vi "Main program.vi"() -> ()   [LabVIEW 2015]
doc: "Use this template to build a standard state machine design pattern. Each state executes code and determines which state to transition to. Contrast this design pattern with the User Interface Event Handler pattern, in which code executes in response to user actions. Contrast this design pattern also with the Queued Message Handler pattern, in which each message handling code can queue zero or more new messages.\nNote: This template does not contain the most recent programming guidelines recommended by National Instruments. For a complete, project-based implementation of the Standard State Machine pattern, use the Create Project dialog box instead of this template."
uses:
  StateMachineStates.ctl
  <vilib>/Analysis/6fits.llb/Curve Fitting Criteria.ctl
  <vilib>/Utility/file.llb/Read From Spreadsheet File (DBL).vi
  <vilib>/Analysis/NI_AALPro.lvlib
panel:
  out "Galv. cal. data":dbl[][](array[numeric])
  out "Galvanostatic":bool
  out "Potentiostatic":bool
  out "DAC calibration data":dbl[][](array[numeric]) format="%0.3f"
  out "Cell on (checkbox)":bool
  out "Current (µA)":dbl format="%.3f"
  in  "Stop button":bool
  out "Voltage (V)":dbl format="%.5f"
  in  "Tab Control":T1(tab)
  in  "Cell on (button)":bool
  in  "Mode":string(combo)="Potentiostatic"
  in  "Current Range":string(combo)="2"
  out "Serial Number":string
  out "Model Name":string
  out "Manufacturer Name":string
  out "Calibrated":bool
  in  "Load DAC calibration":bool
  in  "Scan DAC codes":bool
  out "Code":u16
  in  "DAC output (V)":dbl(slide) scale=0.0..4.8
  out "Config. byte":u8 format="%02x"
  out "Config. byte":u8 format="%02x"
  in  "Calibration factor":dbl=1.0 min=1.0 max=1.0
  in  "ADC CH2 - Current":bool=TRUE
  in  "Bit Depth selection 2":enum32{"CH1", "CH2", "CH2 2", "CH2 3"}(radio)=enum."CH2 3"
  in  "Calibration factor":dbl=3.0
  in  "ADC CH1 - Voltage":bool=TRUE
  in  "Bit Depth selection 1":enum32{"CH1", "CH2", "CH2 2", "CH2 3"}(radio)=enum."CH2 2"
  out "Calibrated 2":bool
  in  "Load galv. calibration":bool
  in  "Calibrate galvanostatic":bool
  in  "VISA resource":refnum<visa-resource-name>
  in  "Auto bit depth":bool
  out "CV graph":cluster{dbl[], dbl[]}(graph)
  in  "Start CV":bool
  in  "Lower bound (V)":dbl=1.0
  in  "Scan rate (mV/s)":dbl=20.0
  in  "Stop CV":bool
  in  "Start potential (V)":dbl=1.0
  in  "Stop potential (V)":dbl=3.0
  in  "Number of cycles":u16
  in  "Upper bound (V)":dbl=3.0
  in  "Copy OCP":bool
  in  "Export filename":path
  in  "Auto range":bool
  out "Calculated capacity values (µAh)":dbl[](array[numeric]) format="%#.4f"
  out "Discharge capacity (µAh)":dbl
  out "Charge capacity (µAh)":dbl
  out "Current half cycle":i32
  in  "Start CC":bool
  in  "Stop CC":bool
  in  "Export filename":path
  in  "Number of\nhalf cycles":u16=3 min=1 step=1
  in  "Copy negative":bool
  in  "Discharge\ncurrent (µA)":dbl=1.0
  in  "Charge\ncurrent (µA)":dbl=1.0
  out "CC ch/disch graph":cluster{dbl[], dbl[]}(graph)
  in  "Upper limit (V)":dbl=3.0
  in  "Lower limit (V)":dbl=1.0
  # "Interface"
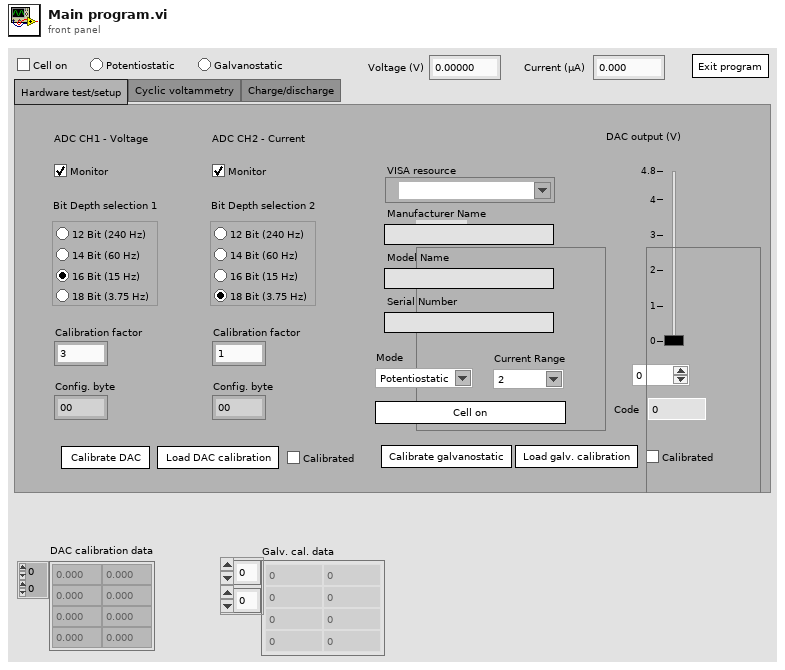
[diagram p1: front panel]
types:
  T1 = enum32{"Hardware test/setup", "Cyclic voltammetry", "Charge/discharge"}
  T2 = typedef "StateMachineStates.ctl" = enum16{"Initialize", "Wait for input", "Perform CV scan", "CC charge/discharge", "Scan DAC codes", "Calibrate galvanostatic", "Stop"}
  T3 = enum16{"open", "replace", "create", "open or create", "replace or create", "replace or create with confirmation"}
  T4 = typedef "NI_AALPro.lvlib/Curve Fitting Criteria.ctl" = u16
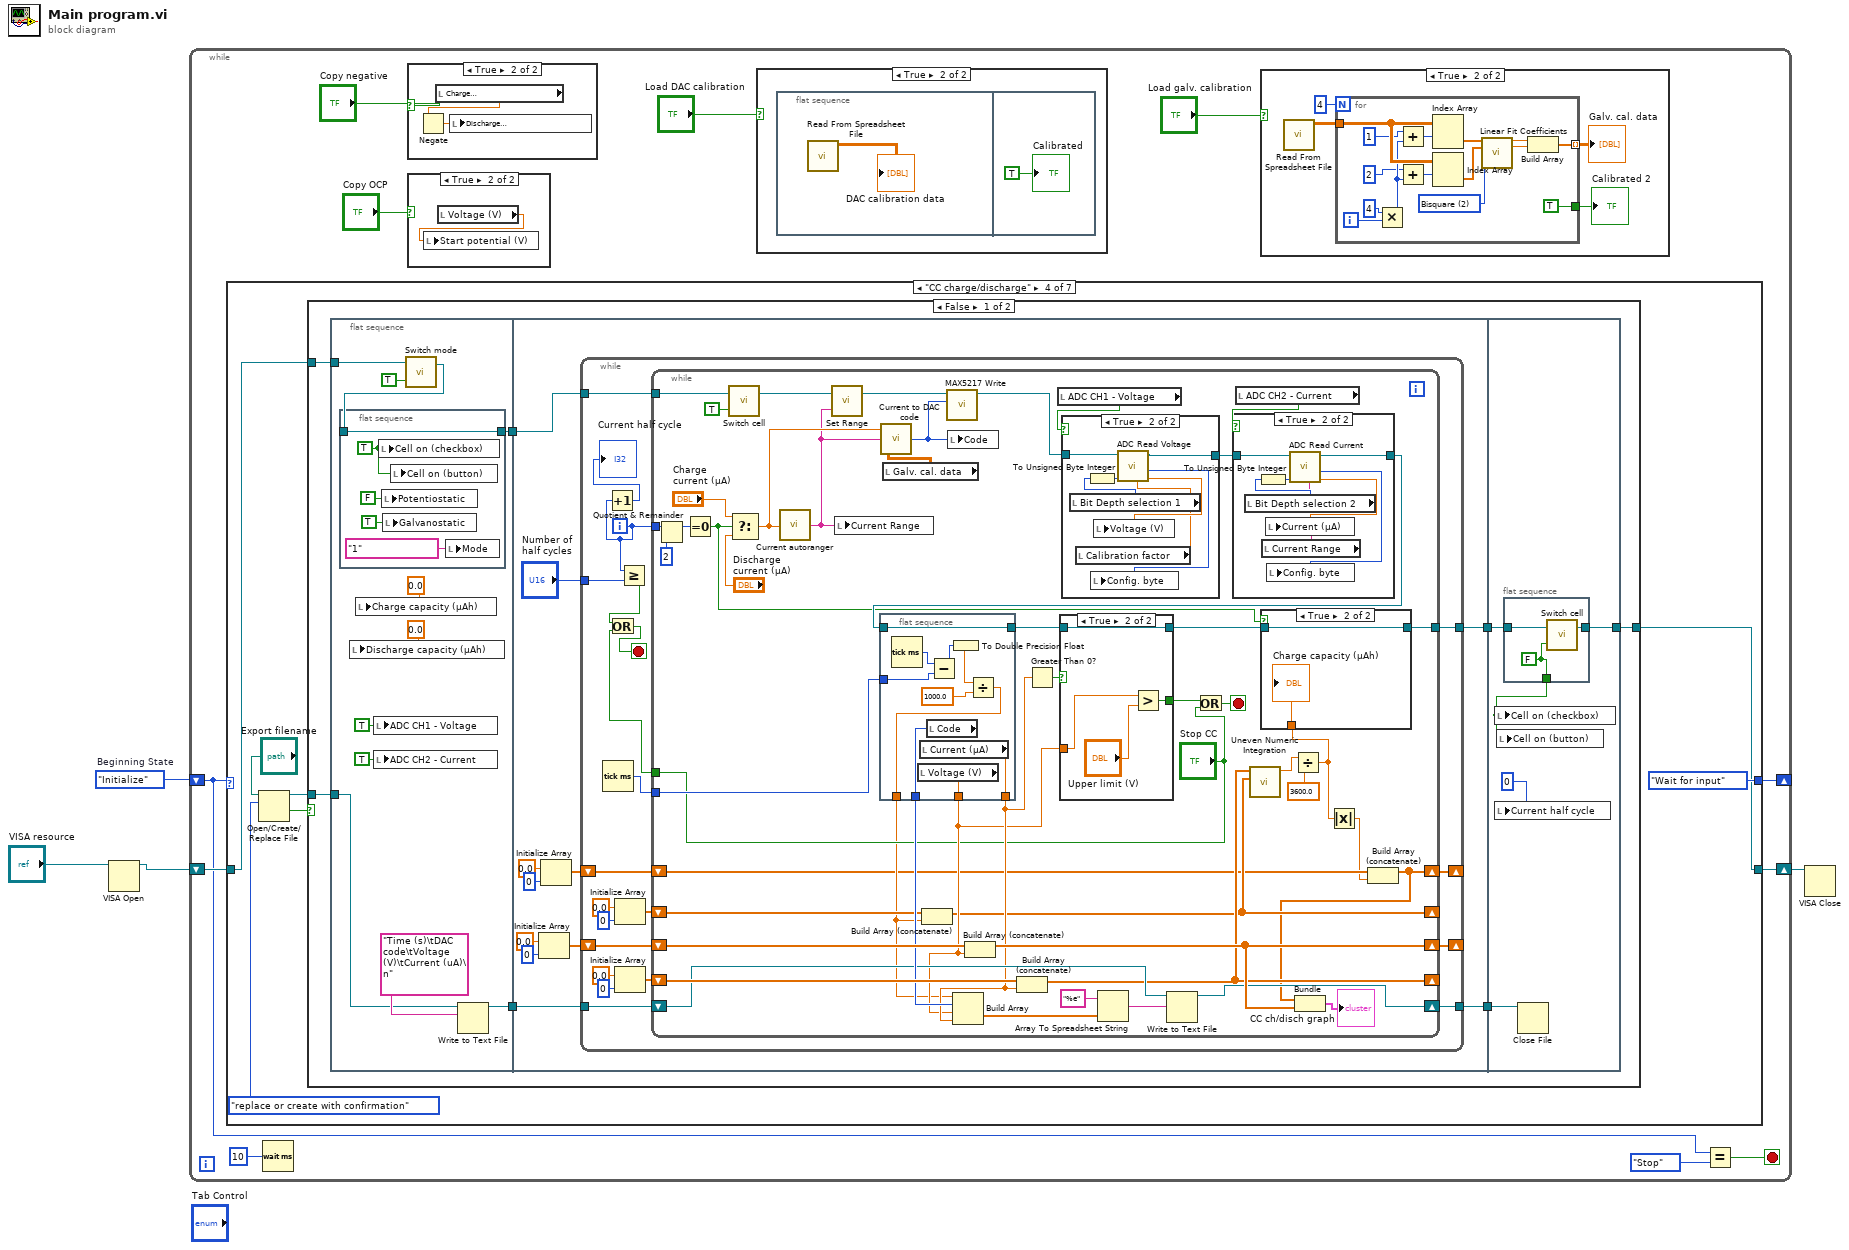
[diagram p0: block diagram]
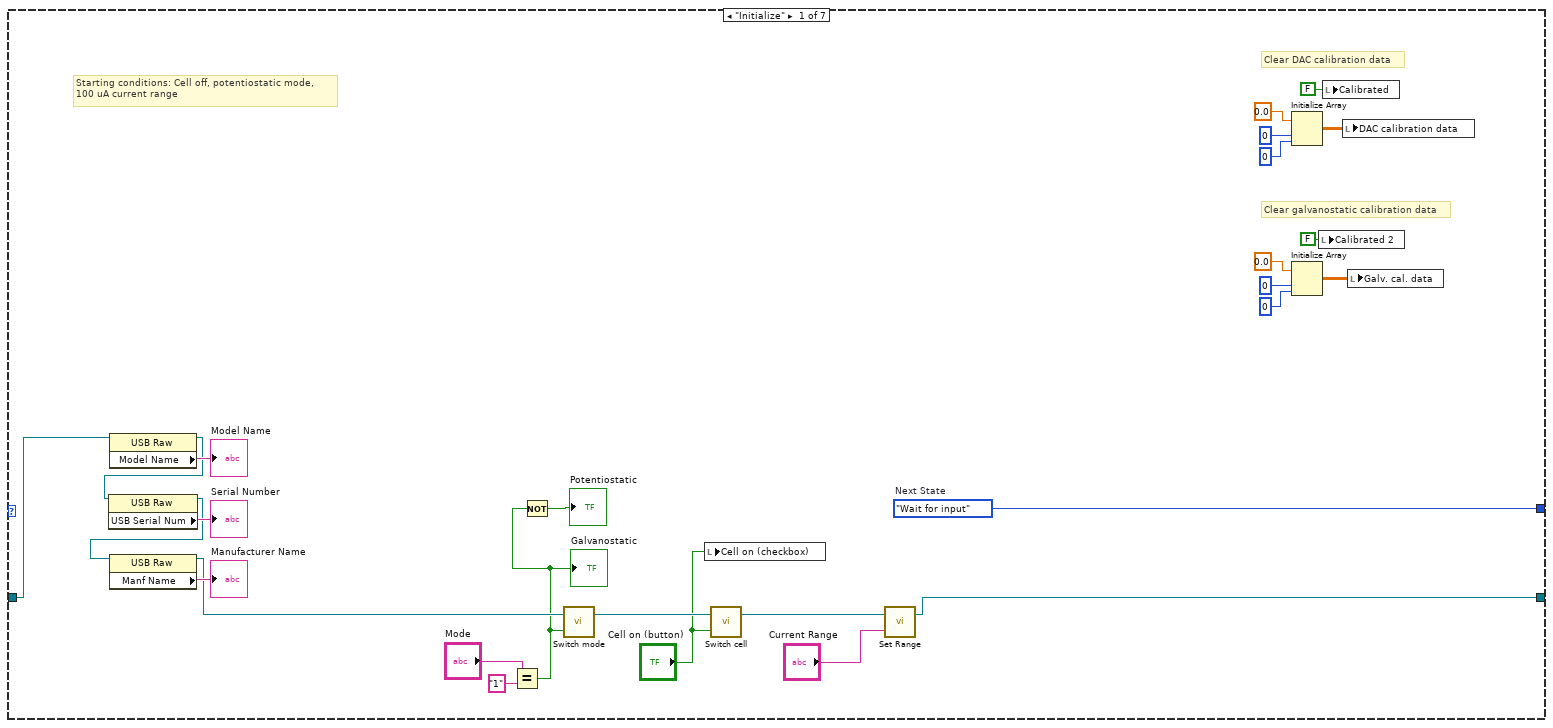
[diagram p6: hidden frame]
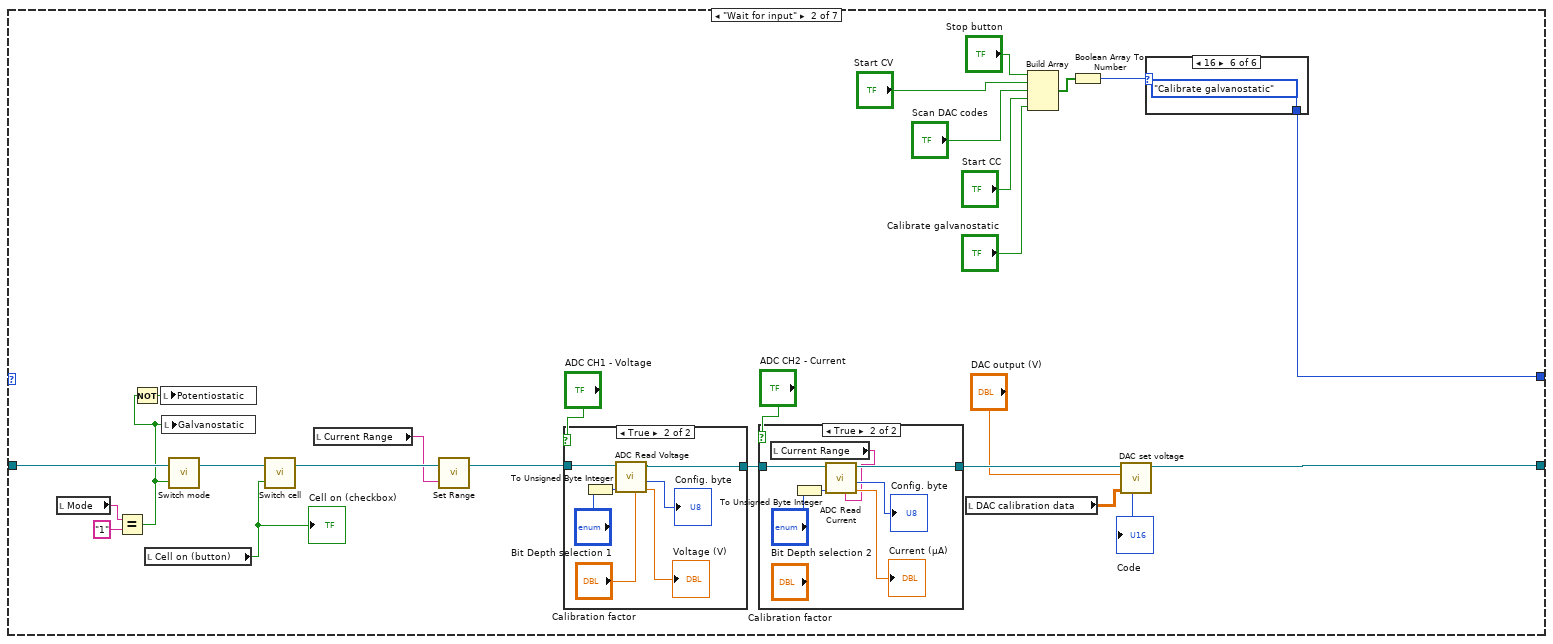
[diagram p7: hidden frame]
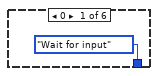
[diagram p10: hidden frame]
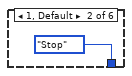
[diagram p11: hidden frame]
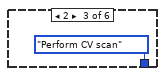
[diagram p12: hidden frame]
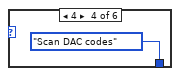
[diagram p13: hidden frame]
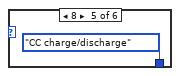
[diagram p14: hidden frame]
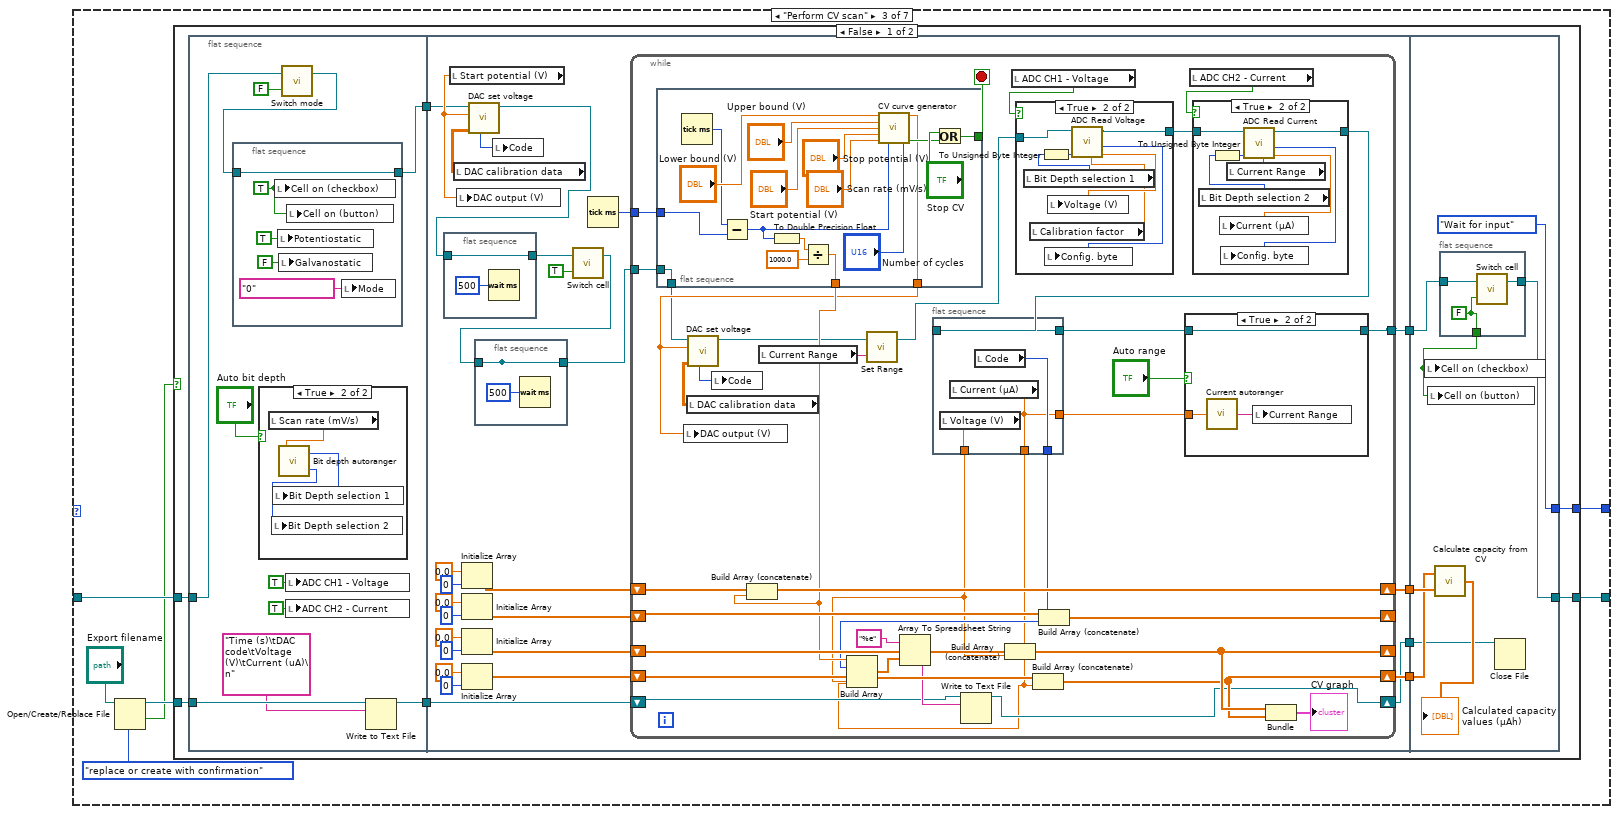
[diagram p15: hidden frame]
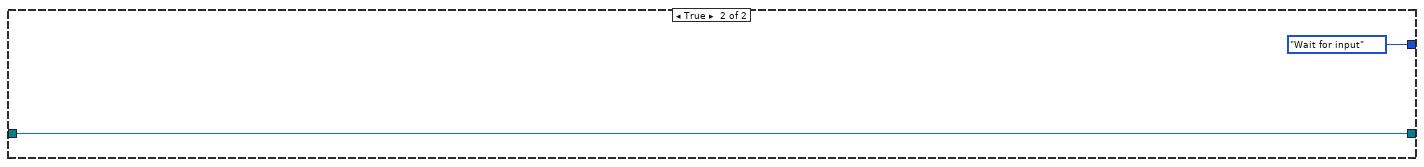
[diagram p20: hidden frame]
diagram:
  w4 = StateMachineStates."Initialize"  # Beginning State
  n1 = VISA Open(VISA resource name="VISA resource") -> (VISA resource name=w1:refnum<visa-resource-name>)  [unwired: 4 in, 1 out]
  n2 = while {
    shift-right: [w14] -> _
    shift-left: w4 -> [w10]
    shift-right: [w11] -> w3
    shift-left: w1 -> [w12]
    stop <- w9 stop-if-true
    n3 = case shown="\"CC charge/discharge\"" w10 {
      tunnel: [w66 w90 w120 StateMachineStates."Wait for input" ("Next State") StateMachineStates."Wait for input" ("Next State") StateMachineStates."Wait for input" ("Next State") StateMachineStates."Stop" ("Next State")] -> w14
      tunnel: w12 -> [w52 w75 w121 w273 w430 w490 w580]
      tunnel: [w40 w83 w119 w271 w429 w491 w580] -> w11
      frame "Initialize" {
        w66 = StateMachineStates."Wait for input"  # Next State
        # "Clear galvanostatic calibration data"
        # "Clear DAC calibration data"
        # "Starting conditions: Cell off, potentiostatic mode,\n100 uA current range"
        n4 = property class="USB Raw"(reference=w52) -> (reference out=w51:refnum<visa-resource-name>, "Model Name"=→"Model Name":string)  [unwired: 1 in, 1 out]
        n5 = property class="USB Raw"(reference=w51) -> (reference out=w50:refnum<visa-resource-name>, "USB Serial Num"=→"Serial Number":string)  [unwired: 1 in, 1 out]
        n6 = property class="USB Raw"(reference=w50) -> (reference out=w48:refnum<visa-resource-name>, "Manf Name"=→"Manufacturer Name":string)  [unwired: 1 in, 1 out]
        n7 = Equal?(x="Mode", y="1") -> (x = y?=w42:bool)
        "Galvanostatic" <- w42
        n8 = Not(x=w42) -> (.not. x?=→"Potentiostatic":bool)
        n9 = call "Switch mode.vi"("Galvanostatic"=w42, "VISA Refnum in"=w48) -> ("VISA Refnum out"=w45:refnum<visa-resource-name>)  [unwired: 1 in]
        n10 = local write "Cell on (checkbox)"("Cell on (button)") -> ()
        n11 = call "Switch cell.vi"("Boolean"="Cell on (button)", "VISA Refnum in"=w45) -> ("VISA Refnum out"=w44:refnum<visa-resource-name>)  [unwired: 1 in]
        n12 = call "Set Range.vi"("Range #"="Current Range", "VISA Refnum in"=w44) -> ("VISA Refnum out"=w40:refnum<visa-resource-name>)  [unwired: 1 in]
        n13 = Initialize Array(0.0 ("element"), 0 ("dimension size"), 0 ("dimension size")) -> (w62:dbl[][])
        n14 = Initialize Array(0.0 ("element"), 0 ("dimension size"), 0 ("dimension size")) -> (w59:dbl[][])
        n15 = local write "Calibrated 2"(FALSE ("Calibrated")) -> ()
        n16 = local write "Calibrated"(FALSE ("Calibrated")) -> ()
        n17 = local write "DAC calibration data"(w62) -> ()
        n18 = local write "Galv. cal. data"(w59) -> ()
      }
      frame "Wait for input" {
        n19 = local read "Mode"() -> (w71:string)
        n20 = Equal?(x=w71, y="1") -> (x = y?=w69:bool)
        n21 = Not(x=w69) -> (.not. x?=w70:bool)
        n22 = local read "Cell on (button)"() -> (w68:bool)
        "Cell on (checkbox)" <- w68
        n23 = local write "Potentiostatic"(w70) -> ()
        n24 = local write "Galvanostatic"(w69) -> ()
        n25 = call "Switch mode.vi"("Galvanostatic"=w69, "VISA Refnum in"=w75) -> ("VISA Refnum out"=w74:refnum<visa-resource-name>)  [unwired: 1 in]
        n26 = call "Switch cell.vi"("Boolean"=w68, "VISA Refnum in"=w74) -> ("VISA Refnum out"=w73:refnum<visa-resource-name>)  [unwired: 1 in]
        n27 = local read "Current Range"() -> (w67:string)
        n28 = call "Set Range.vi"("Range #"=w67, "VISA Refnum in"=w73) -> ("VISA Refnum out"=w72:refnum<visa-resource-name>)  [unwired: 1 in]
        n29 = case shown="True" "ADC CH1 - Voltage" {
          tunnel: [w101 w108] -> w86
          tunnel: w72 -> [w101 w107]
          frame False {
          }
          frame True {
            n30 = To Unsigned Byte Integer(number="Bit Depth selection 1") -> (unsigned 8bit integer=w102:u8)
            n31 = call "ADC Read Voltage.vi"("Calibration factor"="Calibration factor", "Bit depth"=w102, "VISA Refnum in"=w107) -> ("Voltage in V"=→"Voltage (V)":dbl, "Configuration byte"=→"Config. byte":u8, "VISA Refnum out"=w108:refnum<visa-resource-name>)  [unwired: 6 in]
          }
        }
        n32 = case shown="True" "ADC CH2 - Current" {
          tunnel: w86 -> [w93 w100]
          tunnel: [w93 w99] -> w84
          frame False {
          }
          frame True {
            n33 = local read "Current Range"() -> (w94:string)
            n34 = To Unsigned Byte Integer(number="Bit Depth selection 2") -> (unsigned 8bit integer=w97:u8)
            n35 = call "ADC Read Current.vi"("Range"=w94, "Bit depth"=w97, "VISA Refnum in"=w100) -> ("Current in uA"=→"Current (µA)":dbl, "Configuration byte"=→"Config. byte":u8, "VISA Refnum out"=w99:refnum<visa-resource-name>)  [unwired: 6 in]
          }
        }
        n36 = local read "DAC calibration data"() -> (w79:dbl[][])
        n37 = Build Array("Stop button", "Start CV", "Scan DAC codes", "Start CC", "Calibrate galvanostatic") -> (w92:bool[])
        n38 = Boolean Array To Number(Boolean array=w92) -> (number=w91:u32)
        n39 = call "DAC set voltage.vi"("Calibration array"=w79, "DAC output (V)"="DAC output (V)", "VISA Refnum in"=w84) -> ("VISA Refnum out"=w83:refnum<visa-resource-name>, "Output code"=→"Code":u16)  [unwired: 7 in]
        n40 = case shown="16" w91 {
          tunnel: [StateMachineStates."Wait for input" ("f") StateMachineStates."Stop" ("f") StateMachineStates."Perform CV scan" ("f") StateMachineStates."Scan DAC codes" ("f") StateMachineStates."CC charge/discharge" ("f") StateMachineStates."Calibrate galvanostatic" ("f")] -> w90
          frame 0 {
          }
          frame 1, Default {
          }
          frame 2 {
          }
          frame 4 {
          }
          frame 8 {
          }
          frame 16 {
          }
        }
      }
      frame "Perform CV scan" {
        n41 = Open/Create/Replace File(file path (use dialog)="Export filename", operation (0:open)=T3."replace or create with confirmation") -> (refnum out=w116:refnum<file>, cancelled=w115:bool)  [unwired: 4 in, 1 out]
        n42 = case shown="False" w115 {
          tunnel: w121 -> [w128 w270]
          tunnel: [w123 StateMachineStates."Wait for input" ("Next State")] -> w120
          tunnel: [w127 w270] -> w119
          tunnel: w116 -> [w126 _]
          frame False {
            n43 = flat-sequence {
              tunnel: w128 -> [w140]
              tunnel: [w138] -> w131
              tunnel: w126 -> [w134]
              tunnel: [w133] -> w130
              tunnel: w131 -> [w155]
              tunnel: [w163] -> w129
              tunnel: w130 -> [w162]
              tunnel: [w161] -> w125
              tunnel: [w160] -> w124
              tunnel: [w159] -> w122
              tunnel: [w265] -> w127
              tunnel: w129 -> [w264]
              tunnel: w125 -> [w261]
              tunnel: w124 -> [w262]
              tunnel: [StateMachineStates."Wait for input" ("Next State")] -> w123
              tunnel: w122 -> [w259]
              frame #0 {
                n44 = flat-sequence {
                  tunnel: w139 -> [w149]
                  tunnel: [w149] -> w138
                  frame #0 {
                    w146 = TRUE ("Boolean")
                    n45 = local write "Cell on (checkbox)"(w146) -> ()
                    n46 = local write "Potentiostatic"(TRUE ("Potentiostatic")) -> ()
                    n47 = local write "Galvanostatic"(FALSE ("Galvanostatic")) -> ()
                    n48 = local write "Cell on (button)"(w146) -> ()
                    n49 = local write "Mode"("0" ("Mode")) -> ()
                  }
                }
                n50 = case shown="True" "Auto bit depth" {
                  frame False {
                  }
                  frame True {
                    n51 = local read "Scan rate (mV/s)"() -> (w144:dbl)
                    n52 = call "Bit depth autoranger.vi"("Scan rate (mV/s)"=w144) -> ("I bit depth setting"=w142:u8, "V bit depth setting"=w143:u8)  [unwired: 1 in]
                    n53 = local write "Bit Depth selection 2"(w142) -> ()
                    n54 = local write "Bit Depth selection 1"(w143) -> ()
                  }
                }
                n55 = call "Switch mode.vi"("Galvanostatic"=FALSE, "VISA Refnum in"=w140) -> ("VISA Refnum out"=w139:refnum<visa-resource-name>)  [unwired: 1 in]
                n56 = local write "ADC CH1 - Voltage"(TRUE ("ADC CH1 - Voltage")) -> ()
                n57 = local write "ADC CH2 - Current"(TRUE ("ADC CH2 - Current")) -> ()
                n58 = Write to Text File(file (use dialog)=w134, text="Time (s)\tDAC code\tVoltage (V)\tCurrent (uA)\n") -> (refnum out=w133:refnum<file>)  [unwired: 2 in, 2 out]
              }
              frame #1 {
                n59 = flat-sequence {
                  tunnel: [w179] -> w152
                  tunnel: w154 -> [w179]
                  frame #0 {
                    n60 = Wait (ms)(milliseconds to wait=u32 500) -> ()  [unwired: 1 out]
                  }
                }
                n61 = local read "Start potential (V)"() -> (w156:dbl)
                n62 = local read "DAC calibration data"() -> (w157:dbl[][])
                n63 = local write "DAC output (V)"(w156) -> ()
                n64 = Initialize Array(0.0 ("element"), 0 ("dimension size")) -> (w167:dbl[])
                n65 = Initialize Array(0.0 ("element"), 0 ("dimension size")) -> (w164:dbl[])
                n66 = Initialize Array(0.0 ("element"), 0 ("dimension size")) -> (w175:dbl[])
                n67 = Initialize Array(0.0 ("element"), 0 ("dimension size")) -> (w172:dbl[])
                n68 = call "DAC set voltage.vi"("Calibration array"=w157, "DAC output (V)"=w156, "VISA Refnum in"=w155) -> ("VISA Refnum out"=w154:refnum<visa-resource-name>, "Output code"=w158:u16)  [unwired: 7 in]
                n69 = flat-sequence {
                  tunnel: [w177] -> _
                  tunnel: w151 -> [w177]
                  tunnel: [w177] -> w150
                  frame #0 {
                    n70 = Wait (ms)(milliseconds to wait=u32 500) -> ()  [unwired: 1 out]
                  }
                }
                n71 = local write "Code"(w158) -> ()
                n72 = call "Switch cell.vi"("Boolean"=TRUE, "VISA Refnum in"=w152) -> ("VISA Refnum out"=w151:refnum<visa-resource-name>)  [unwired: 1 in]
                n73 = Tick Count (ms)() -> (millisecond timer value=w176:u32)
                n74 = while {
                  tunnel: w176 -> [w208]
                  tunnel: w150 -> [w204]
                  tunnel: [w189] -> w163
                  shift-right: [w214] -> _
                  shift-left: w175 -> [w216]
                  shift-right: [w213] -> w161
                  shift-left: w172 -> [w215]
                  shift-right: [w210] -> w160
                  shift-left: w167 -> [w209]
                  shift-right: [w203] -> _
                  shift-left: w164 -> [w202]
                  shift-right: [w191] -> w159
                  shift-left: w162 -> [w192]
                  stop <- w211 stop-if-true
                  n75 = flat-sequence {
                    tunnel: [w241] -> w211
                    tunnel: w208 -> [w231]
                    tunnel: [w227] -> w196
                    tunnel: w204 -> [w225]
                    tunnel: [w226] -> w184
                    tunnel: [w225] -> w183
                    frame #0 {
                      n76 = Tick Count (ms)() -> (millisecond timer value=w232:u32)
                      n77 = Subtract(x=w232, y=w231) -> (x-y=w229:u32)
                      n78 = To Double Precision Float(number=w229) -> (double precision float=w228:dbl)
                      n79 = Divide(x=w228, y=1000.0) -> (x/y=w227:dbl)
                      n80 = call "CV curve generator.vi"("Lower bound (V)"="Lower bound (V)", "Upper bound (V)"="Upper bound (V)", "Start potential (V)"="Start potential (V)", "Stop potential (V)"="Stop potential (V)", "Scan rate (mV/s)"="Scan rate (mV/s)", "Time (ms)"=w229, "Number of cycles"="Number of cycles") -> ("Actual potential"=w226:dbl, "End"=w233:bool)  [unwired: 7 in]
                      n81 = Or(x="Stop CV", y=w233) -> (x .or. y?=w241:bool)
                    }
                  }
                  n82 = local write "DAC output (V)"(w184) -> ()
                  n83 = local read "DAC calibration data"() -> (w199:dbl[][])
                  n84 = call "DAC set voltage.vi"("Calibration array"=w199, "DAC output (V)"=w184, "VISA Refnum in"=w183) -> ("VISA Refnum out"=w182:refnum<visa-resource-name>, "Output code"=w200:u16)  [unwired: 7 in]
                  n85 = local write "Code"(w200) -> ()
                  n86 = Build Array (concatenate)(w209, w196) -> (w210:dbl[])
                  n87 = local read "Current Range"() -> (w185:string)
                  n88 = Build Array(w196, w195, w194, w186) -> (w197:dbl[])
                  n89 = call "Set Range.vi"("Range #"=w185, "VISA Refnum in"=w182) -> ("VISA Refnum out"=w181:refnum<visa-resource-name>)  [unwired: 1 in]
                  n90 = Array To Spreadsheet String(array=w197, 3:"%e" ("format string")) -> (spreadsheet string=w193:string)  [unwired: 1 out]
                  n91 = flat-sequence {
                    tunnel: w201 -> [w222]
                    tunnel: [w224] -> w194
                    tunnel: [w221] -> w186
                    tunnel: [w223] -> w195
                    tunnel: [w222] -> w190
                    tunnel: [w221] -> w187
                    frame #0 {
                      n92 = local read "Voltage (V)"() -> (w224:dbl)
                      n93 = local read "Current (µA)"() -> (w221:dbl)
                      n94 = local read "Code"() -> (w223:u16)
                    }
                  }
                  n95 = Write to Text File(file (use dialog)=w192, text=w193) -> (refnum out=w191:refnum<file>)  [unwired: 2 in, 2 out]
                  n96 = Build Array (concatenate)(w216, w194) -> (w214:dbl[])
                  n97 = local read "ADC CH1 - Voltage"() -> (w206:bool)
                  n98 = case shown="True" w206 {
                    tunnel: [w250 w257] -> w207
                    tunnel: w181 -> [w250 w256]
                    frame False {
                    }
                    frame True {
                      n99 = local read "Bit Depth selection 1"() -> (w254:enum32{"CH1", "CH2", "CH2 2", "CH2 3"})
                      n100 = local read "Calibration factor"() -> (w252:dbl)
                      n101 = To Unsigned Byte Integer(number=w254) -> (unsigned 8bit integer=w255:u8)
                      n102 = call "ADC Read Voltage.vi"("Calibration factor"=w252, "Bit depth"=w255, "VISA Refnum in"=w256) -> ("Voltage in V"=w253:dbl, "Configuration byte"=w251:u8, "VISA Refnum out"=w257:refnum<visa-resource-name>)  [unwired: 6 in]
                      n103 = local write "Config. byte"(w251) -> ()
                      n104 = local write "Voltage (V)"(w253) -> ()
                    }
                  }
                  n105 = Build Array (concatenate)(w215, w186) -> (w213:dbl[])
                  n106 = Build Array (concatenate)(w202, w195) -> (w203:dbl[])
                  n107 = case shown="True" "Auto range" {
                    tunnel: w190 -> [w217 w220]
                    tunnel: [w217 w220] -> w189
                    tunnel: w187 -> [_ w219]
                    frame False {
                    }
                    frame True {
                      n108 = call "Current autoranger.vi"("Current (µA)"=w219) -> ("Range"=w218:string)
                      n109 = local write "Current Range"(w218) -> ()
                    }
                  }
                  n110 = local read "ADC CH2 - Current"() -> (w205:bool)
                  n111 = case shown="True" w205 {
                    tunnel: w207 -> [w242 w249]
                    tunnel: [w242 w248] -> w201
                    frame False {
                    }
                    frame True {
                      n112 = local read "Bit Depth selection 2"() -> (w246:enum32{"CH1", "CH2", "CH2 2", "CH2 3"})
                      n113 = To Unsigned Byte Integer(number=w246) -> (unsigned 8bit integer=w247:u8)
                      n114 = local read "Current Range"() -> (w243:string)
                      n115 = call "ADC Read Current.vi"("Range"=w243, "Bit depth"=w247, "VISA Refnum in"=w249) -> ("Current in uA"=w245:dbl, "Configuration byte"=w244:u8, "VISA Refnum out"=w248:refnum<visa-resource-name>)  [unwired: 6 in]
                      n116 = local write "Current (µA)"(w245) -> ()
                      n117 = local write "Config. byte"(w244) -> ()
                    }
                  }
                  n118 = Bundle(w214, w213) -> (→"CV graph":cluster{dbl[], dbl[]})  [unwired: 1 in]
                }
              }
              frame #2 {
                n119 = local write "Cell on (checkbox)"(w258) -> ()
                n120 = local write "Cell on (button)"(w258) -> ()
                n121 = call "Calculate capacity from CV.vi"("t values"=w262, "I values"=w261) -> ("Capacity values"=→"Calculated capacity values (µAh)":dbl[])  [unwired: 1 in]
                n122 = flat-sequence {
                  tunnel: w264 -> [w268]
                  tunnel: [w267] -> w265
                  tunnel: [w266] -> w258
                  frame #0 {
                    w266 = FALSE ("Boolean")
                    n123 = call "Switch cell.vi"("Boolean"=w266, "VISA Refnum in"=w268) -> ("VISA Refnum out"=w267:refnum<visa-resource-name>)  [unwired: 1 in]
                  }
                }
                n124 = Close File(refnum=w259) -> ()  [unwired: 1 in, 2 out]
              }
            }
          }
          frame True {
          }
        }
      }
      frame "CC charge/discharge" {
        n125 = Open/Create/Replace File(file path (use dialog)="Export filename", operation (0:open)=T3."replace or create with confirmation") -> (refnum out=w272:refnum<file>, cancelled=w274:bool)  [unwired: 4 in, 1 out]
        n126 = case shown="False" w274 {
          tunnel: w273 -> [w284 w428]
          tunnel: w272 -> [w283 _]
          tunnel: [w279 w428] -> w271
          frame False {
            n127 = flat-sequence {
              tunnel: w284 -> [w294]
              tunnel: w283 -> [w289]
              tunnel: [w288] -> w282
              tunnel: [w287] -> w281
              tunnel: w282 -> [w310]
              tunnel: w281 -> [w311]
              tunnel: [w309] -> w280
              tunnel: [w304] -> w278
              tunnel: w280 -> [w424]
              tunnel: [w423] -> w279
              tunnel: w278 -> [w421]
              frame #0 {
                n128 = flat-sequence {
                  tunnel: w293 -> [w300]
                  tunnel: [w300] -> w287
                  frame #0 {
                    w297 = TRUE ("Boolean")
                    n129 = local write "Cell on (checkbox)"(w297) -> ()
                    n130 = local write "Potentiostatic"(FALSE ("Potentiostatic")) -> ()
                    n131 = local write "Galvanostatic"(TRUE ("Galvanostatic")) -> ()
                    n132 = local write "Cell on (button)"(w297) -> ()
                    n133 = local write "Mode"("1" ("Mode")) -> ()
                  }
                }
                n134 = local write "Discharge capacity (µAh)"(0.0 ("Discharge capacity (µAh)")) -> ()
                n135 = local write "Charge capacity (µAh)"(0.0 ("Charge capacity (µAh)")) -> ()
                n136 = local write "ADC CH1 - Voltage"(TRUE ("ADC CH1 - Voltage")) -> ()
                n137 = local write "ADC CH2 - Current"(TRUE ("ADC CH2 - Current")) -> ()
                n138 = call "Switch mode.vi"("Galvanostatic"=TRUE ("Potentiostatic"), "VISA Refnum in"=w294) -> ("VISA Refnum out"=w293:refnum<visa-resource-name>)  [unwired: 1 in]
                n139 = Write to Text File(file (use dialog)=w289, text="Time (s)\tDAC code\tVoltage (V)\tCurrent (uA)\n") -> (refnum out=w288:refnum<file>)  [unwired: 2 in, 2 out]
              }
              frame #1 {
                n140 = Initialize Array(0.0 ("element"), 0 ("dimension size")) -> (w306:dbl[])
                n141 = Initialize Array(0.0 ("element"), 0 ("dimension size")) -> (w301:dbl[])
                n142 = while {
                  tunnel: w311 -> [w332]
                  tunnel: w310 -> [w331]
                  tunnel: [w329] -> w309
                  shift-right: [w324] -> _
                  shift-left: w306 -> [w325]
                  tunnel: "Number of\nhalf cycles" -> [w323]
                  tunnel: [w314] -> w304
                  shift-right: [w312] -> _
                  shift-left: w301 -> [w313]
                  i -> [w322]
                  stop <- w328 stop-if-true
                  n143 = Tick Count (ms)() -> (millisecond timer value=w330:u32)
                  n144 = Increment(x=w322) -> (x+1=→"Current half cycle":i32)
                  n145 = Initialize Array(0.0 ("element"), 0 ("dimension size")) -> (w315:dbl[])
                  n146 = Initialize Array(0.0 ("element"), 0 ("dimension size")) -> (w318:dbl[])
                  n147 = Greater Or Equal?(x=w322, y=w323) -> (x >= y?=w327:bool)
                  n148 = while {
                    tunnel: w322 -> [w379]
                    tunnel: w332 -> [w335]
                    shift-right: [w364] -> w314
                    shift-left: w331 -> [w365]
                    tunnel: w330 -> [w367]
                    tunnel: [w349] -> w329
                    tunnel: ["Stop CC"] -> w326
                    shift-right: [w371] -> w324
                    shift-left: w325 -> [w374]
                    shift-right: [w352] -> _
                    shift-left: w318 -> [w373]
                    shift-right: [w351] -> _
                    shift-left: w315 -> [w354]
                    shift-right: [w343] -> w312
                    shift-left: w313 -> [w345]
                    stop <- w359 stop-if-true
                    n149 = Quotient & Remainder(x=w379, y=2) -> (x-y*floor(x/y)=w381:i32)  [unwired: 1 out]
                    n150 = Equal To 0?(x=w381) -> (x = 0?=w348:bool)
                    n151 = call "Switch cell.vi"("Boolean"=TRUE, "VISA Refnum in"=w335) -> ("VISA Refnum out"=w334:refnum<visa-resource-name>)  [unwired: 1 in]
                    n152 = Select(t="Charge\ncurrent (µA)", s=w348, f="Discharge\ncurrent (µA)") -> (s? t:f=w342:dbl)
                    n153 = call "Current autoranger.vi"("Current (µA)"=w342) -> ("Range"=w336:string)
                    n154 = call "Set Range.vi"("Range #"=w336, "VISA Refnum in"=w334) -> ("VISA Refnum out"=w337:refnum<visa-resource-name>)  [unwired: 1 in]
                    n155 = local write "Current Range"(w336) -> ()
                    n156 = flat-sequence {
                      tunnel: w375 -> [w394]
                      tunnel: [w403] -> w360
                      tunnel: [w402] -> w368
                      tunnel: [w397] -> w353
                      tunnel: [w396] -> w362
                      tunnel: w367 -> [w395]
                      tunnel: [w394] -> w361
                      frame #0 {
                        n157 = Tick Count (ms)() -> (millisecond timer value=w401:u32)
                        n158 = local read "Voltage (V)"() -> (w403:dbl)
                        n159 = local read "Current (µA)"() -> (w396:dbl)
                        n160 = local read "Code"() -> (w402:u16)
                        n161 = Subtract(x=w401, y=w395) -> (x-y=w400:u32)
                        n162 = To Double Precision Float(number=w400) -> (double precision float=w399:dbl)
                        n163 = Divide(x=w399, y=1000.0) -> (x/y=w397:dbl)
                      }
                    }
                    n164 = local read "Galv. cal. data"() -> (w341:dbl[][])
                    n165 = call "Current to DAC code.vi"("Galv. cal. data"=w341, "Current Range"=w336, "DAC output (µA)"=w342) -> ("Code out"=w339:u16)
                    n166 = Build Array (concatenate)(w354, w353) -> (w351:dbl[])
                    n167 = call "MAX5217 Write.vi"("DAC code"=w339, "VISA Refnum in"=w337) -> ("VISA Refnum out"=w338:refnum<visa-resource-name>)  [unwired: 6 in, 1 out]
                    n168 = local write "Code"(w339) -> ()
                    n169 = Build Array(w353, w368, w360, w362) -> (w370:dbl[])
                    n170 = Build Array (concatenate)(w374, w360) -> (w371:dbl[])
                    n171 = Build Array (concatenate)(w373, w362) -> (w352:dbl[])
                    n172 = Greater Than 0?(x=w362) -> (x > 0?=w363:bool)
                    n173 = local read "ADC CH1 - Voltage"() -> (w377:bool)
                    n174 = case shown="True" w363 {
                      tunnel: w361 -> [w386 w393]
                      tunnel: [w386 w393] -> w350
                      tunnel: w360 -> [w387 w392]
                      tunnel: [w389 w390] -> w358
                      frame False {
                        n175 = Less?(x=w387, y="Lower limit (V)") -> (x < y?=w389:bool)
                      }
                      frame True {
                        n176 = Greater?(x=w392, y="Upper limit (V)") -> (0:w390:bool)
                      }
                    }
                    n177 = case shown="True" w377 {
                      tunnel: [w412 w419] -> w378
                      tunnel: w338 -> [w412 w418]
                      frame False {
                      }
                      frame True {
                        n178 = local read "Bit Depth selection 1"() -> (w416:enum32{"CH1", "CH2", "CH2 2", "CH2 3"})
                        n179 = local read "Calibration factor"() -> (w414:dbl)
                        n180 = To Unsigned Byte Integer(number=w416) -> (unsigned 8bit integer=w417:u8)
                        n181 = call "ADC Read Voltage.vi"("Calibration factor"=w414, "Bit depth"=w417, "VISA Refnum in"=w418) -> ("Voltage in V"=w415:dbl, "Configuration byte"=w413:u8, "VISA Refnum out"=w419:refnum<visa-resource-name>)  [unwired: 6 in]
                        n182 = local write "Config. byte"(w413) -> ()
                        n183 = local write "Voltage (V)"(w415) -> ()
                      }
                    }
                    n184 = Array To Spreadsheet String(array=w370, 3:"%e" ("format string")) -> (spreadsheet string=w366:string)  [unwired: 1 out]
                    n185 = Write to Text File(file (use dialog)=w365, text=w366) -> (refnum out=w364:refnum<file>)  [unwired: 2 in, 2 out]
                    n186 = Or(x=w358, y="Stop CC") -> (x .or. y?=w359:bool)
                    n187 = local read "ADC CH2 - Current"() -> (w376:bool)
                    n188 = case shown="True" w376 {
                      tunnel: w378 -> [w404 w411]
                      tunnel: [w404 w410] -> w375
                      frame False {
                      }
                      frame True {
                        n189 = local read "Bit Depth selection 2"() -> (w408:enum32{"CH1", "CH2", "CH2 2", "CH2 3"})
                        n190 = To Unsigned Byte Integer(number=w408) -> (unsigned 8bit integer=w409:u8)
                        n191 = local read "Current Range"() -> (w405:string)
                        n192 = call "ADC Read Current.vi"("Range"=w405, "Bit depth"=w409, "VISA Refnum in"=w411) -> ("Current in uA"=w407:dbl, "Configuration byte"=w406:u8, "VISA Refnum out"=w410:refnum<visa-resource-name>)  [unwired: 6 in]
                        n193 = local write "Current (µA)"(w407) -> ()
                        n194 = local write "Config. byte"(w406) -> ()
                      }
                    }
                    n195 = call <vilib>:"Uneven Numeric Integration.vi"("T"=w351, "X"=w352) -> ("result"=w346:dbl)  [unwired: 8 in, 1 out]
                    n196 = Divide(x=w346, y=3600.0) -> (x/y=w344:dbl)
                    n197 = case shown="True" w348 {
                      tunnel: w350 -> [w382 w385]
                      tunnel: [w382 w385] -> w349
                      tunnel: w344 -> [w383 w384]
                      frame False {
                        "Discharge capacity (µAh)" <- w383
                      }
                      frame True {
                        "Charge capacity (µAh)" <- w384
                      }
                    }
                    n198 = Absolute Value(x=w344) -> (abs(x)=w340:dbl)
                    n199 = Build Array (concatenate)(w345, w340) -> (w343:dbl[])
                    n200 = Bundle(w343, w371) -> (→"CC ch/disch graph":cluster{dbl[], dbl[]})  [unwired: 1 in]
                  }
                  n201 = Or(x=w327, y=w326) -> (x .or. y?=w328:bool)
                }
              }
              frame #2 {
                n202 = local write "Cell on (checkbox)"(w420) -> ()
                n203 = local write "Current half cycle"(0 ("Current half cycle")) -> ()
                n204 = local write "Cell on (button)"(w420) -> ()
                n205 = flat-sequence {
                  tunnel: w424 -> [w425]
                  tunnel: [w427] -> w423
                  tunnel: [w426] -> w420
                  frame #0 {
                    w426 = FALSE ("Boolean")
                    n206 = call "Switch cell.vi"("Boolean"=w426, "VISA Refnum in"=w425) -> ("VISA Refnum out"=w427:refnum<visa-resource-name>)  [unwired: 1 in]
                  }
                }
                n207 = Close File(refnum=w421) -> ()  [unwired: 1 in, 2 out]
              }
            }
          }
          frame True {
          }
        }
      }
      frame "Scan DAC codes" {
        n208 = Two Button Dialog(message="This procedure will scan all possible output codes of the DAC (ranging from 0 to 65535) and record the resulting voltage as a function of the DAC code in a two-column ASCII text file. This will take a long time. Make sure that the electrodes are disconnected.") -> (T button?=w431:bool)  [unwired: 2 in]
        n209 = case shown="True" w431 {
          tunnel: [w434 w439] -> w429
          tunnel: w430 -> [w434 w440]
          frame False {
          }
          frame True {
            n210 = Open/Create/Replace File(prompt="Choose or enter a filename to save the DAC calibration file", operation (0:open)=T3."replace or create") -> (refnum out=w436:refnum<file>, cancelled=w437:bool)  [unwired: 4 in, 1 out]
            n211 = case shown="False" w437 {
              tunnel: w440 -> [w443 w489]
              tunnel: [w448 w489] -> w439
              tunnel: w436 -> [w447 _]
              frame False {
                w441 = FALSE ("Boolean")
                n212 = flat-sequence {
                  tunnel: w445 -> [w456]
                  tunnel: [w455] -> w444
                  frame #0 {
                    w451 = TRUE ("Boolean")
                    n213 = local write "Cell on (checkbox)"(w451) -> ()
                    n214 = local write "Potentiostatic"(TRUE ("Potentiostatic")) -> ()
                    n215 = local write "Galvanostatic"(FALSE ("Galvanostatic")) -> ()
                    n216 = local write "Cell on (button)"(w451) -> ()
                    n217 = call "Switch cell.vi"("Boolean"=w451, "VISA Refnum in"=w456) -> ("VISA Refnum out"=w455:refnum<visa-resource-name>)  [unwired: 1 in]
                    n218 = local write "Mode"("0" ("Mode")) -> ()
                  }
                }
                n219 = call "Switch mode.vi"("Galvanostatic"=FALSE ("Potentiostatic"), "VISA Refnum in"=w443) -> ("VISA Refnum out"=w445:refnum<visa-resource-name>)  [unwired: 1 in]
                n220 = while {
                  tunnel: [w473] -> w450
                  tunnel: w444 -> [w472]
                  tunnel: [w457] -> w449
                  shift-right: [w462] -> w442
                  shift-left: w447 -> [w463]
                  i -> [w461]
                  stop <- w471 stop-if-true
                  n221 = flat-sequence {
                    tunnel: w472 -> [w477]
                    tunnel: w461 -> [w475]
                    tunnel: [w476] -> w467
                    tunnel: [w474] -> w458
                    tunnel: w467 -> [w482]
                    tunnel: [w482] -> w466
                    tunnel: w458 -> [w480]
                    tunnel: w466 -> [w488]
                    tunnel: [w487] -> w457
                    tunnel: [w484] -> w460
                    frame #0 {
                      n222 = To Unsigned Word Integer(number=w475) -> (unsigned 16bit integer=w474:u16)
                      n223 = call "MAX5217 Write.vi"("DAC code"=w474, "VISA Refnum in"=w477) -> ("VISA Refnum out"=w476:refnum<visa-resource-name>)  [unwired: 6 in, 1 out]
                    }
                    frame #1 {
                      n224 = Equal?(x=u16 0, y=w480) -> (x = y?=w478:bool)
                      n225 = case shown="True" w478 {
                        frame False {
                        }
                        frame True {
                          n226 = Wait (ms)(milliseconds to wait=u32 5000) -> ()  [unwired: 1 out]
                        }
                      }
                      n227 = Wait (ms)(milliseconds to wait=u32 100) -> ()  [unwired: 1 out]
                    }
                    frame #2 {
                      n228 = local read "Calibration factor"() -> (w485:dbl)
                      n229 = call "ADC Read Voltage.vi"("Calibration factor"=w485, "Bit depth"=u8 3, "VISA Refnum in"=w488) -> ("Voltage in V"=w484:dbl, "VISA Refnum out"=w487:refnum<visa-resource-name>)  [unwired: 6 in, 1 out]
                    }
                  }
                  n230 = Build Array(w461, w460) -> (w459:dbl[])
                  n231 = Array To Spreadsheet String(array=w459, 3:"%e" ("format string")) -> (spreadsheet string=w465:string)  [unwired: 1 out]
                  n232 = Write to Text File(file (use dialog)=w463, text=w465) -> (refnum out=w462:refnum<file>)  [unwired: 2 in, 2 out]
                  n233 = call "Progress bar DAC scan.vi"("Voltage (V)"=w460, "DAC code"=w461) -> ("Abort"=w470:bool, "Prog Bar Ref"=w473:refnum<vi>)
                  n234 = Greater Or Equal?(x=w461, y=65535) -> (x >= y?=w469:bool)
                  n235 = Or(x=w470, y=w469) -> (x .or. y?=w471:bool)
                }
                n236 = local write "Cell on (checkbox)"(w441) -> ()
                n237 = local write "Cell on (button)"(w441) -> ()
                n238 = Close File(refnum=w442) -> ()  [unwired: 1 in, 2 out]
                n239 = invoke class="VI" method="FP.Close"(reference=w450) -> ()  [unwired: 2 in, 3 out]
                n240 = call "Switch cell.vi"("Boolean"=w441, "VISA Refnum in"=w449) -> ("VISA Refnum out"=w448:refnum<visa-resource-name>)  [unwired: 1 in]
              }
              frame True {
              }
            }
          }
        }
      }
      frame "Calibrate galvanostatic" {
        n241 = Two Button Dialog(message="This procedure will record the cell current as a function of the voltage sent to the galvanostatic control loop. This will take some time. Please short the electrodes before starting the procedure.") -> (T button?=w493:bool)  [unwired: 2 in]
        n242 = case shown="True" w493 {
          tunnel: [w495 w500] -> w491
          tunnel: w490 -> [w495 w501]
          frame False {
          }
          frame True {
            n243 = Open/Create/Replace File(prompt="Choose or enter a filename to save the galvanostatic calibration file", operation (0:open)=T3."replace or create") -> (refnum out=w497:refnum<file>, cancelled=w498:bool)  [unwired: 4 in, 1 out]
            n244 = case shown="False" w498 {
              tunnel: w501 -> [w511 w579]
              tunnel: [w513 w579] -> w500
              tunnel: w497 -> [w506 _]
              frame False {
                n245 = flat-sequence {
                  tunnel: w504 -> [w521]
                  tunnel: [w520] -> w503
                  frame #0 {
                    w516 = TRUE ("Boolean")
                    n246 = local write "Cell on (checkbox)"(w516) -> ()
                    n247 = local write "Potentiostatic"(FALSE ("Potentiostatic")) -> ()
                    n248 = local write "Galvanostatic"(TRUE ("Galvanostatic")) -> ()
                    n249 = local write "Cell on (button)"(w516) -> ()
                    n250 = call "Switch cell.vi"("Boolean"=w516, "VISA Refnum in"=w521) -> ("VISA Refnum out"=w520:refnum<visa-resource-name>)  [unwired: 1 in]
                    n251 = local write "Mode"("1" ("Mode")) -> ()
                  }
                }
                n252 = call "Switch mode.vi"("Galvanostatic"=TRUE ("Potentiostatic"), "VISA Refnum in"=w511) -> ("VISA Refnum out"=w504:refnum<visa-resource-name>)  [unwired: 1 in]
                n253 = for {
                  N: 4 -> [_]
                  tunnel: [w537] -> w515
                  tunnel: [w536] -> w514
                  tunnel: w503 -> [w526]
                  tunnel: [w527] -> w507 mode=indexing
                  i -> [w523]
                  n254 = Initialize Array(u16 0 ("element"), 0 ("dimension size")) -> (w533:u16[])
                  n255 = Initialize Array(0.0 ("element"), 0 ("dimension size")) -> (w530:dbl[])
                  n256 = Increment(x=w523) -> (x+1=w522:i32)
                  n257 = Number To Decimal String(number=w522) -> (decimal integer string=w524:string)  [unwired: 1 in]
                  n258 = call "Set Range.vi"("Range #"=w524, "VISA Refnum in"=w526) -> ("VISA Refnum out"=w525:refnum<visa-resource-name>)  [unwired: 1 in]
                  n259 = while {
                    tunnel: [w544] -> w537
                    tunnel: w525 -> [w545]
                    tunnel: [w553] -> w536
                    shift-right: [w550] -> w529
                    shift-left: w533 -> [w549]
                    shift-right: [w548] -> w528
                    shift-left: w530 -> [w547]
                    tunnel: w522 -> [w538]
                    tunnel: w524 -> [w539]
                    i -> [w546]
                    stop <- w557 stop-if-true
                    n260 = flat-sequence {
                      tunnel: [w559] -> w551
                      tunnel: w546 -> [w563]
                      tunnel: w545 -> [w560]
                      tunnel: [w562] -> w540
                      tunnel: [w569] -> w554
                      tunnel: [w567] -> w552
                      tunnel: w551 -> [w567]
                      tunnel: w540 -> [w569]
                      tunnel: w554 -> [w575]
                      tunnel: [w574] -> w553
                      tunnel: [w572] -> w541
                      tunnel: [w571] -> w542
                      tunnel: w552 -> [w571]
                      tunnel: w539 -> [w570]
                      frame #0 {
                        n261 = To Unsigned Word Integer(number=w563) -> (unsigned 16bit integer=w564:u16)
                        n262 = Increment(x=w564) -> (x+1=w565:u16)
                        n263 = Multiply(x=w565, y=u16 1000) -> (x*y=w561:u16)
                        n264 = Add(x=u16 500, y=w561) -> (x+y=w559:u16)
                        n265 = call "MAX5217 Write.vi"("DAC code"=w559, "VISA Refnum in"=w560) -> ("VISA Refnum out"=w562:refnum<visa-resource-name>)  [unwired: 6 in, 1 out]
                      }
                      frame #1 {
                        n266 = Wait (ms)(milliseconds to wait=u32 5000) -> ()  [unwired: 1 out]
                      }
                      frame #2 {
                        n267 = call "ADC Read Current.vi"("Range"=w570, "Bit depth"=u8 3, "VISA Refnum in"=w575) -> ("Current in uA"=w572:dbl, "VISA Refnum out"=w574:refnum<visa-resource-name>)  [unwired: 6 in, 1 out]
                      }
                    }
                    n268 = Greater Or Equal?(x=w546, y=10) -> (x >= y?=w556:bool)
                    n269 = Build Array (concatenate)(w549, w542) -> (w550:u16[])
                    n270 = Build Array (concatenate)(w547, w541) -> (w548:dbl[])
                    n271 = call "Progress bar galvanostatic calibration.vi"("Range #"=w538, "Current (µA)"=w541, "DAC code"=w542) -> ("Abort"=w543:bool, "Prog Bar Ref"=w544:refnum<vi>)
                    n272 = Or(x=w543, y=w556) -> (x .or. y?=w557:bool)
                  }
                  n273 = Build Array(w529, w528) -> (w527:dbl[][])
                }
                n274 = invoke class="VI" method="FP.Close"(reference=w515) -> ()  [unwired: 2 in, 3 out]
                n275 = local write "Cell on (checkbox)"(w502) -> ()
                n276 = local write "Cell on (button)"(w502) -> ()
                n277 = flat-sequence {
                  tunnel: w514 -> [w578]
                  tunnel: [w577] -> w513
                  tunnel: [w576] -> w502
                  frame #0 {
                    w576 = FALSE ("Boolean")
                    n278 = call "Switch cell.vi"("Boolean"=w576, "VISA Refnum in"=w578) -> ("VISA Refnum out"=w577:refnum<visa-resource-name>)  [unwired: 1 in]
                  }
                }
                n279 = Array To Spreadsheet String(array=w507, 3:"%e" ("format string")) -> (spreadsheet string=w508:string)  [unwired: 1 out]
                n280 = Write to Text File(file (use dialog)=w506, text=w508) -> (refnum out=w505:refnum<file>)  [unwired: 2 in, 2 out]
                n281 = Close File(refnum=w505) -> ()  [unwired: 1 in, 2 out]
              }
              frame True {
              }
            }
          }
        }
      }
      frame "Stop" {
      }
    }
    n282 = Wait (ms)(milliseconds to wait=u32 10) -> ()  [unwired: 1 out]
    n283 = case shown="True" "Copy negative" {
      frame False {
      }
      frame True {
        n284 = local read "Charge\ncurrent (µA)"() -> (w35:dbl)
        n285 = Negate(x=w35) -> (-x=w36:dbl)
        n286 = local write "Discharge\ncurrent (µA)"(w36) -> ()
      }
    }
    n287 = case shown="True" "Copy OCP" {
      frame False {
      }
      frame True {
        n288 = local read "Voltage (V)"() -> (w39:dbl)
        n289 = local write "Start potential (V)"(w39) -> ()
      }
    }
    n290 = case shown="True" "Load DAC calibration" {
      frame False {
      }
      frame True {
        n291 = flat-sequence {
          frame #0 {
            n292 = call-poly <vilib>:"Read From Spreadsheet File.vi"() -> ("all rows"=→"DAC calibration data":dbl[][])  [unwired: 7 in, 4 out]
          }
          frame #1 {
            "Calibrated" <- TRUE ("DAC calibrated")
          }
        }
      }
    }
    n293 = case shown="True" "Load galv. calibration" {
      frame False {
      }
      frame True {
        n294 = call-poly <vilib>:"Read From Spreadsheet File.vi"() -> ("all rows"=w19:dbl[][])  [unwired: 7 in, 4 out]
        n295 = for {
          N: 4 -> [_]
          tunnel: w19 -> [w34]
          tunnel: [w22] -> w17 mode=indexing
          tunnel: [TRUE ("DAC calibrated")] -> w16
          i -> [w29]
          w20 = T4 2 items=["Least Square", "Least Absolute Residual", "Bisquare"] ("method")
          n296 = Multiply(x=4, y=w29) -> (x*y=w24:i32)
          n297 = Add(x=1 ("index (row)"), y=w24) -> (x+y=w27:i32)
          n298 = Add(x=2 ("index (row)"), y=w24) -> (x+y=w25:i32)
          n299 = Index Array(array=w34, index (row)=w27) -> (element=w33:dbl[])  [unwired: 1 in]
          n300 = Index Array(array=w34, index (row)=w25) -> (element=w32:dbl[])  [unwired: 1 in]
          n301 = call <vilib>:"Linear Fit Coefficients.vi"("Y"=w33, "X"=w32, "method"=w20) -> ("slope"=w31:dbl, "intercept"=w30:dbl)  [unwired: 10 in, 1 out]
          n302 = Build Array(w31, w30) -> (w22:dbl[])
        }
        "Galv. cal. data" <- w17
        "Calibrated 2" <- w16
      }
    }
    n303 = Equal?(x=w10, y=StateMachineStates."Stop" ("States")) -> (x = y?=w9:bool)
  }
  n304 = VISA Close(VISA resource name=w3) -> ()  [unwired: 1 in, 1 out]
